vi "ShowDataSub.vi"(11 "SubChannel in":refnum<class "SubChannelCPU.lvclass">) -> (0 "elements":cluster{"elt":T1}[](array[cluster]), 1 "size":i32, 2 "count":i32, 3 "SubChannel out":refnum<class "SubChannelCPU.lvclass">, 4 "unbounded":bool, 6 "active":bool, 8 "last element":bool)   [LabVIEW 2019, in "MessengerM.lvlib" / "SubChannelCPU.lvclass"]
uses:
  SubChannelCPU.lvclass
  <resource>/ChannelSupport/_ChannelSupport/PipeLogic2/PipeLogic2.lvclass
  Element.ctl
  MessengerM.lvlib
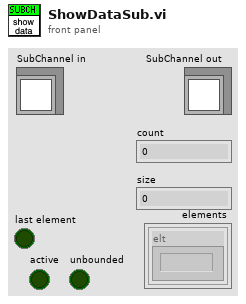
[diagram p1: front panel]
types:
  T1 = typedef "MessengerM.lvlib/Element.ctl" = string
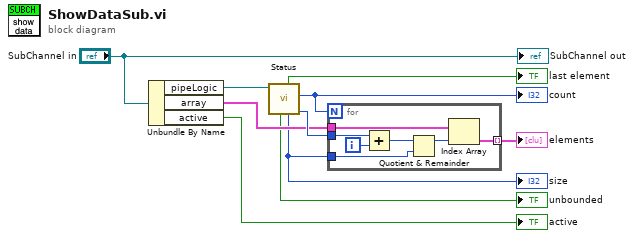
[diagram p0: block diagram]
diagram:
  n1 = Unbundle By Name("SubChannel in") -> ("pipeLogic"=w8:refnum<class "PipeLogic2.lvclass">, "array"=w7:cluster{"elt":T1}[], "active"=→"active":bool)
  n2 = call <resource>:"Status.vi"("pipeLogic in"=w8) -> ("index out"=w9:i32, "count"=w3:i32, "size"=w5:i32, "last element"=→"last element":bool, "unbounded"=→"unbounded":bool)  [unwired: 4 in, 2 out]
  "count" <- w3
  "size" <- w5
  n3 = for {
    N: w3 -> [_]
    tunnel: w7 -> [w17]
    tunnel: w9 -> [w16]
    tunnel: [w12] -> w6 mode=indexing
    tunnel: w5 -> [w11]
    i -> [w15]
    n4 = Add(x=w16, y=w15) -> (x+y=w14:i32)
    n5 = Quotient & Remainder(x=w14, y=w11) -> (x-y*floor(x/y)=w13:i32)  [unwired: 1 out]
    n6 = Index Array(array=w17, index=w13) -> (element=w12:cluster{"elt":T1})
  }
  "elements" <- w6
  "SubChannel out" <- "SubChannel in"
